vi "Test Set Cell Font.vi"(11 "Test Case In":refnum<class "Test Open Xml.lvclass">) -> (0 "error out":errorcluster, 3 "Test Case Out":refnum<class "Test Open Xml.lvclass">)   [LabVIEW 2020, in "Test Open Xml.lvclass"]
uses:
  Test Open Xml.lvclass
  <vilib>/Astemes/LUnit/Test Case.lvclass
  Source/Open Xml.lvlib
  4b527410-3829-466b-86c3-b8d1fd0707f5.vi
  Source/Font.ctl
  2693d141-7dae-43f3-880c-0f0d59430732.vi
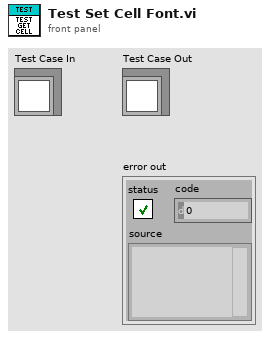
[diagram p1: front panel]
types:
  T1 = typedef "Open Xml.lvlib/Font.ctl" = cluster{"Bold":enum16{"bold", "regular", "default"}, "Italic":enum16{"italic", "regular", "default"}, "Underline":enum16{"single", "double", "singleAccounting", "doubleAccounting", "none", "default"}, "TextColor":u32, "TextSize":dbl, "Name":string}
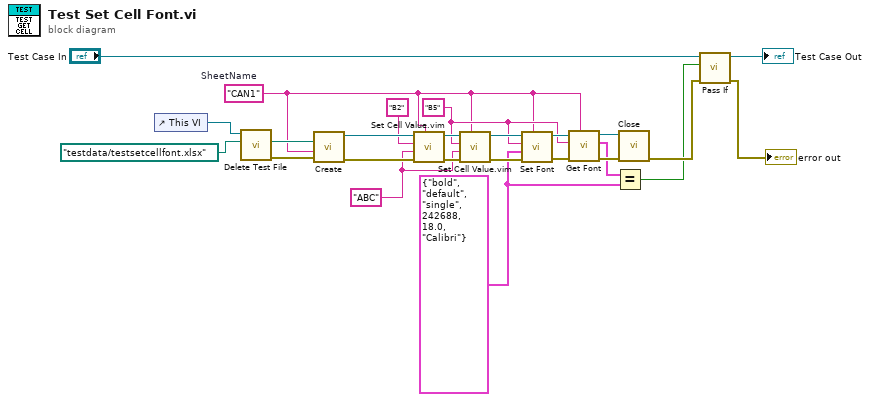
[diagram p0: block diagram]
diagram:
  w1 = "ABC" ("Value")
  w13 = T1 {"Bold"=enum."bold", "Italic"=enum."default", "Underline"=enum."single", "TextColor"=242688, "TextSize"=18.0, "Name"="Calibri"} ("Font")
  w4 = "B5" ("Cell Address")
  w2 = "CAN1"  # SheetName
  n1 = control-ref of="This VI"() -> (w10:refnum<vi>)
  n2 = call "Delete Test File.vi"("name or relative path"=path "testdata/testsetcellfont.xlsx", "VI in"=w10) -> ("error out"=w9:errorcluster, "deleted path"=w8:path)  [unwired: 8 in]
  n3 = call "Create.vi"("error in"=w9, "SheetName"=w2, "Path"=w8) -> ("error out"=w22:errorcluster, "SpreadsheetDoc"=w6:refnum<k24>)  [unwired: 7 in]
  n4 = call "Set Cell Value.vim"("Sheet Name"=w2, "error in"=w22, "Value"=w1, "Cell Address"="B2", "SpreadsheetDoc in"=w6) -> ("error out"=w7:errorcluster, "SpreadsheetDoc out"=w5:refnum<k24>)  [unwired: 5 in]
  n5 = call "Set Cell Value.vim"("Sheet Name"=w2, "error in"=w7, "Value"=w1, "Cell Address"=w4, "SpreadsheetDoc in"=w5) -> ("error out"=w20:errorcluster, "SpreadsheetDoc out"=w18:refnum<k24>)  [unwired: 5 in]
  n6 = call "Set Font.vi"("Sheet Name"=w2, "error in"=w20, "Font"=w13, "Cell Address"=w4, "SpreadsheetDoc in"=w18) -> ("error out"=w19:errorcluster, "SpreadsheetDoc out"=w16:refnum<k24>)  [unwired: 5 in]
  n7 = call "Get Font.vi"("Sheet Name"=w2, "error in"=w19, "Cell Address"=w4, "SpreadsheetDoc in"=w16) -> ("error out"=w17:errorcluster, "Font"=w14:T1, "SpreadsheetDoc out"=w15:refnum<k24>)  [unwired: 5 in]
  n8 = Equal?(x=w14, y=w13) -> (x = y?=w12:bool)
  n9 = call "Close.vi"("error in"=w17, "SpreadsheetDoc"=w15) -> ("error out"=w21:errorcluster)  [unwired: 9 in]
  n10 = call <vilib>:"Pass If.vi"("error in (no error)"=w21, "Pass?"=w12, "LUnit Test Case In"="Test Case In") -> ("error out"=→"error out":errorcluster, "LUnit Test Case Out"=→"Test Case Out":refnum<class "Test Open Xml.lvclass">)  [unwired: 7 in]
